vi "SWERVE_DRIVE_BEGIN.vi"(8 "error in (no error)":errorcluster) -> (0 "error out":errorcluster, 1 "Init Gyro Value":dbl, 2 "Swerve Module Pos":T1[](array[typedef]) {"Angle"."SIN" format="%13.4f"; "Angle"."COS" format="%13.4f"; "Angle"."VALUE" format="%13.4f"}, 3 "SWERVE_DRIVE_KINEMATICS":T3 {"SavedModuleStates"."Angle"."SIN" format="%13.4f"; "SavedModuleStates"."Angle"."COS" format="%13.4f"; "SavedModuleStates"."Angle"."VALUE" format="%13.4f"; "PrevCoR"."Y" format="%14.3f"; "PrevCoR"."X" format="%14.3f"; "Modules"."Y" format="%14.3f"; "Modules"."X" format="%14.3f"})   [LabVIEW 2019]
uses:
  <vilib>/Rock Robotics/WPI/ThirdParty/JAS_Junk/TrajLib/TypeDef/SWERVE_DRIVE_KINEMATICS.ctl
  <vilib>/Analysis/Matrix/Datatypes/RealMatrix.ctl
  <vilib>/Rock Robotics/WPI/ThirdParty/JAS_Junk/TrajLib/TypeDef/TRANSLATION2D.ctl
  <vilib>/Rock Robotics/WPI/ThirdParty/JAS_Junk/TrajLib/TypeDef/SWERVE_DRIVE_MODULE_STATE.ctl
  <vilib>/Rock Robotics/WPI/ThirdParty/JAS_Junk/TrajLib/TypeDef/ROTATION2D.ctl
  <vilib>/Rock Robotics/SystemInterfaces/AI/FPGA_AIGyroChannel.ctl
  <vilib>/Rock Robotics/SystemInterfaces/DIO/FPGA_DIOPWMChannel.ctl
  <vilib>/Rock Robotics/SystemInterfaces/DIO/FPGA_DIOChannel.ctl
  <vilib>/Rock Robotics/WPI/Gyro/WPI_GyroAnalogOpen.vi
  <vilib>/Rock Robotics/WPI/ThirdParty/JAS_Junk/TrajLib/Trajectory_Library.lvlib
  <vilib>/Analysis/Matrix/NI_Matrix.lvlib
  <vilib>/Rock Robotics/WPI/ThirdParty/JAS_Junk/TrajLib/TypeDef/SWERVE_DRIVE_MODULE_POSITION.ctl
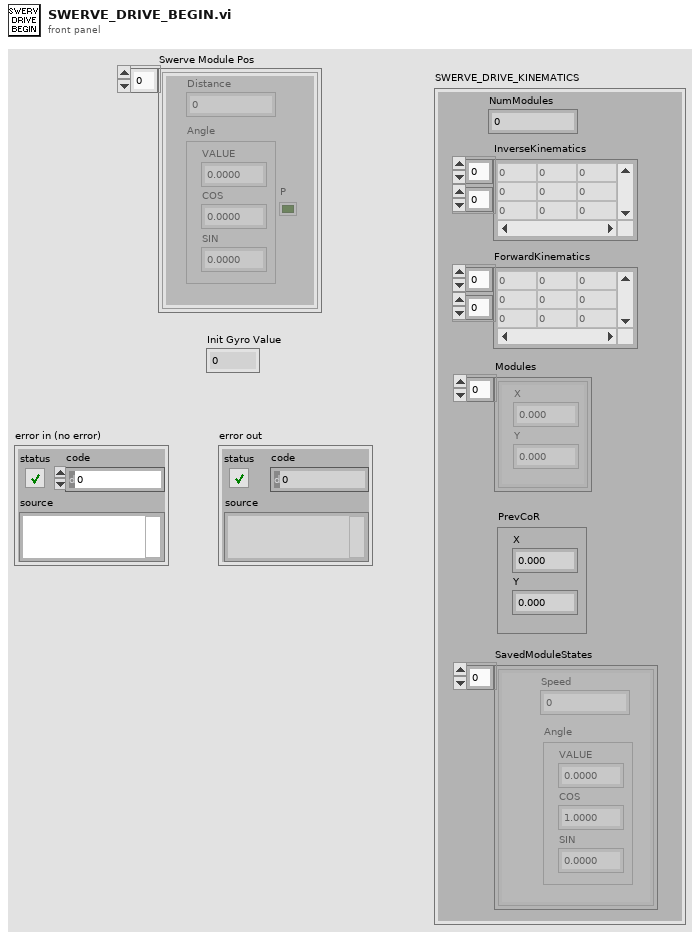
[diagram p1: front panel]
types:
  T1 = typedef "Trajectory_Library.lvlib/SWERVE_DRIVE_MODULE_POSITION.ctl" = cluster{"Distance":dbl, "Angle":T2, "P":bool}
  T2 = typedef "Trajectory_Library.lvlib/ROTATION2D.ctl" = cluster{"VALUE":dbl, "COS":dbl, "SIN":dbl}
  T3 = typedef "Trajectory_Library.lvlib/SWERVE_DRIVE_KINEMATICS.ctl" = cluster{"NumModules":i32, "InverseKinematics":T4, "ForwardKinematics":T4, "Modules":T5[], "PrevCoR":T5, "SavedModuleStates":T6[]}
  T4 = typedef "NI_Matrix.lvlib/RealMatrix.ctl" = dbl[][]
  T5 = typedef "Trajectory_Library.lvlib/TRANSLATION2D.ctl" = cluster{"X":dbl, "Y":dbl}
  T6 = typedef "Trajectory_Library.lvlib/SWERVE_DRIVE_MODULE_STATE.ctl" = cluster{"Speed":dbl, "Angle":T2}
  T7 = typedef "FPGA_DIOChannel.ctl" = enum8{"DIO 0", "DIO 1", "DIO 2", "DIO 3", "DIO 4", "DIO 5", "DIO 6", "DIO 7", "DIO 8", "DIO 9", "DIO MXP 0", "DIO MXP 1", "DIO MXP 2", "DIO MXP 3", "DIO MXP 4", "DIO MXP 5", "DIO MXP 6", "DIO MXP 7", "DIO MXP 8", "DIO MXP 9", "DIO MXP 10", "DIO MXP 11", "DIO MXP 12", "DIO MXP 13", "DIO MXP 14", "DIO MXP 15", "SPI Port CS1", "SPI Port CS2", "SPI Port CS3", "SPI Port MISO", "SPI Port MOSI", "Invalid"}
  T8 = typedef "FPGA_DIOPWMChannel.ctl" = enum8{"PWM 0", "PWM 1", "PWM 2", "PWM 3", "PWM 4", "PWM 5", "PWM 6", "PWM 7", "PWM 8", "PWM 9", "PWM MXP 0", "PWM MXP 1", "PWM MXP 2", "PWM MXP 3", "PWM MXP 4", "PWM MXP 5", "PWM MXP 6", "PWM MXP 7", "PWM MXP 8", "PWM MXP 9", "Invalid"}
  T9 = typedef "FPGA_AIGyroChannel.ctl" = enum8{"AI 0", "AI 1", "Invalid"}
  T10 = typedef "WPI_GyroDevRef.ctl" = cluster{"DevStatus":errorcluster, "Analog Channel":T11, "Gain (VoltsPerDegree/Second)":dbl, "Gyro Type":enum16{"Analog", "XRS450"}, "Handle":i32, "SPI Bus":T12, "Device Found":bool, "Sample Rate":dbl, "Calibrate On Open":bool, "Offset":dbl}
  T11 = typedef "FPGA_AIChannel.ctl" = enum8{"AI 0", "AI 1", "AI 2", "AI 3", "AI MXP 0", "AI MXP 1", "AI MXP 2", "AI MXP 3", "Invalid"}
  T12 = typedef "spi_bus.ctl" = enum16{"SPI On-Board, CS0", "SPI On-Board, CS1", "SPI On-Board, CS2", "SPI On-Board, CS3", "SPI MXP", "Invalid"}
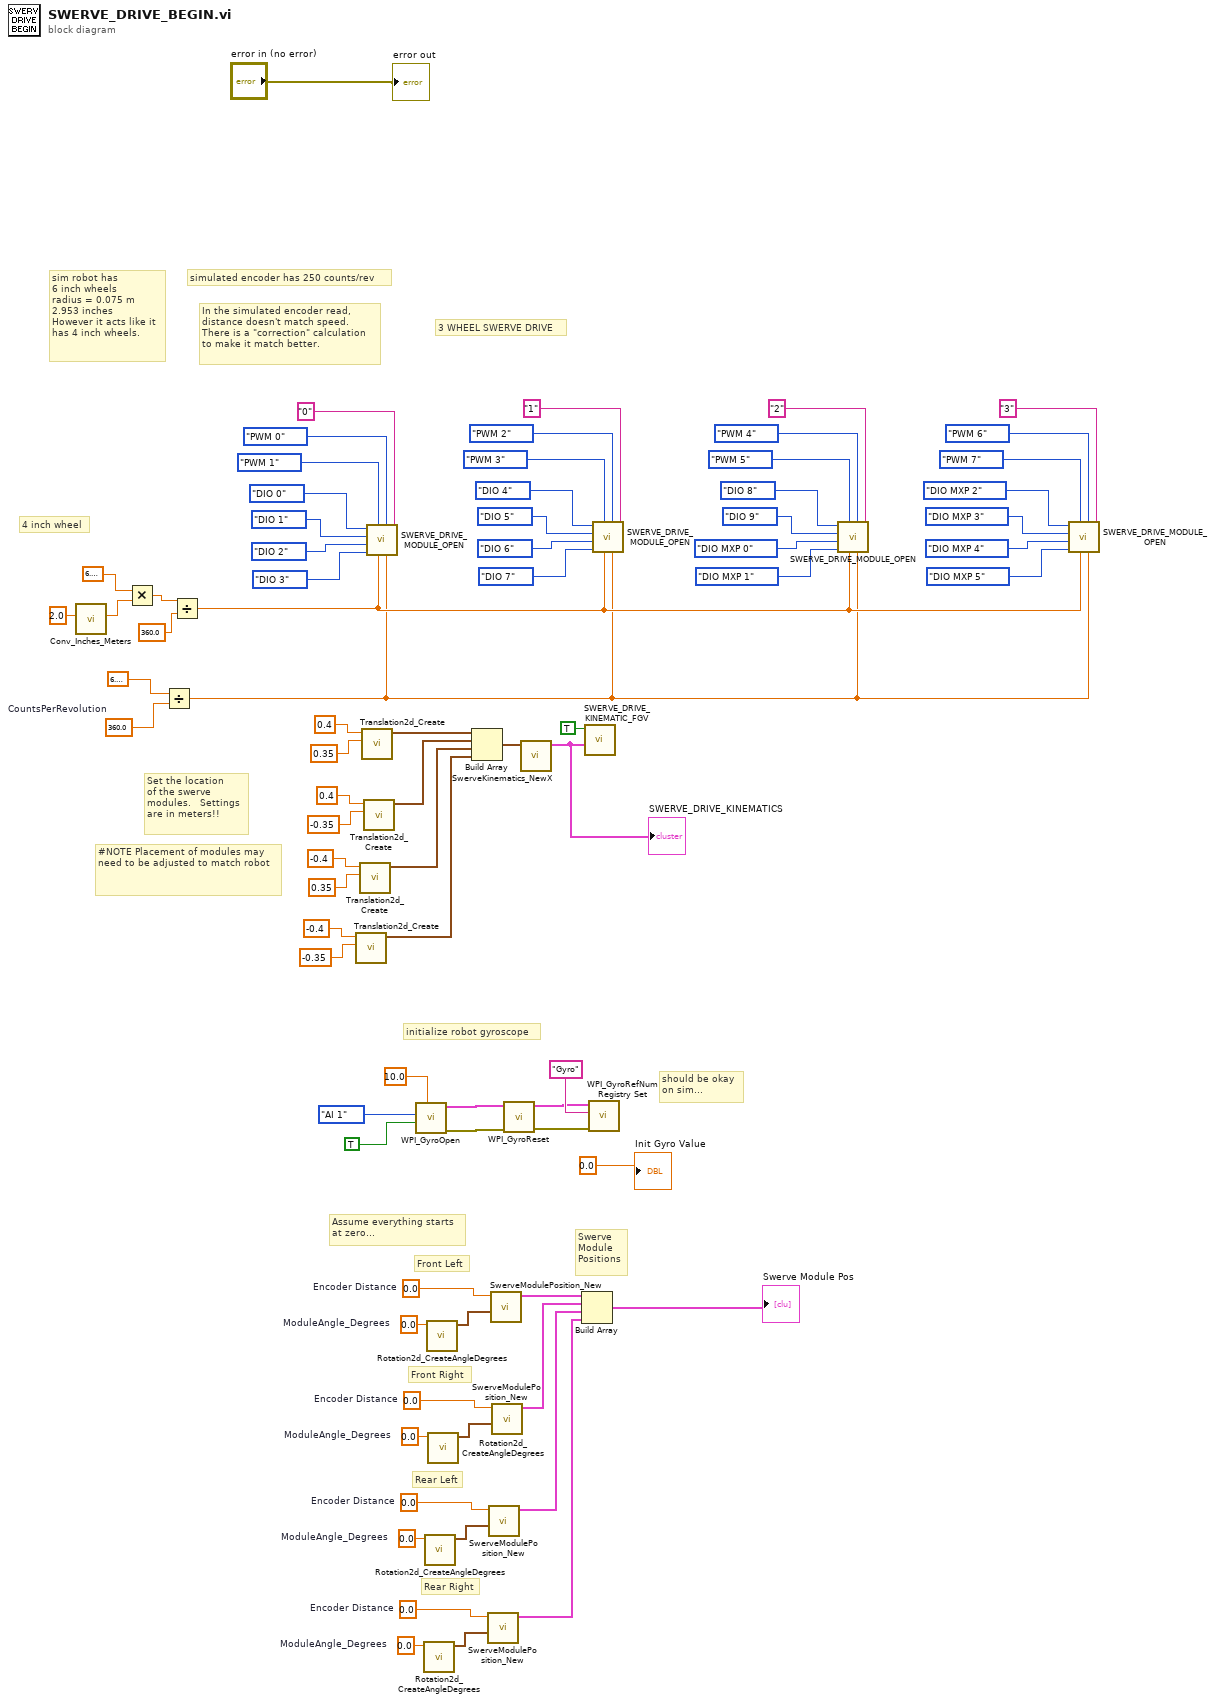
[diagram p0: block diagram]
diagram:
  w19 = 0.0  # ModuleAngle_Degrees
  w17 = 0.0  # Encoder Distance
  w16 = 0.0  # ModuleAngle_Degrees
  w14 = 0.0  # Encoder Distance
  w13 = 0.0  # ModuleAngle_Degrees
  w11 = 0.0  # Encoder Distance
  w9 = 0.0  # ModuleAngle_Degrees
  w7 = 0.0  # Encoder Distance
  w39 = 360.0  # CountsPerRevolution
  # "Assume everything starts\nat zero..."
  # "Front Left"
  # "Swerve\nModule\nPositions"
  # "Rear Right"
  # "Rear Left"
  # "Front Right"
  # "#NOTE Placement of modules may need to be adjusted to match robot"
  # "should be okay\non sim..."
  # "Set the location\nof the swerve \nmodules.   Settings\nare in meters!!"
  # "4 inch wheel"
  # "3 WHEEL SWERVE DRIVE"
  # "initialize robot gyroscope"
  # "In the simulated encoder read,\ndistance doesn't match speed.\nThere is a \"correction\" calculation\nto make it match better."
  # "simulated encoder has 250 counts/rev"
  # "sim robot has\n6 inch wheels\nradius = 0.075 m\n2.953 inches\nHowever it acts like it\nhas 4 inch wheels."
  n1 = call <vilib>:"Conv_Inches_Meters.vi"("INCH"=2.0) -> ("Meters"=w66:dbl)  [unwired: 10 in]
  n2 = Multiply(x=6.283185307179586, y=w66) -> (x*y=w25:dbl)
  n3 = Divide(x=6.283185307179586, y=w39) -> (x/y=w75:dbl)
  n4 = Divide(x=w25, y=360.0) -> (x/y=w76:dbl)
  n5 = call <vilib>:"Translation2d_Create.vi"("Y"=-0.35, "X"=-0.4) -> ("TRANSLATION"=w79:T5)  [unwired: 9 in]
  n6 = call <vilib>:"Translation2d_Create.vi"("Y"=0.35, "X"=-0.4) -> ("TRANSLATION"=w62:T5)  [unwired: 9 in]
  n7 = call <vilib>:"Translation2d_Create.vi"("Y"=0.35, "X"=0.4) -> ("TRANSLATION"=w60:T5)  [unwired: 9 in]
  n8 = call <vilib>:"Translation2d_Create.vi"("Y"=-0.35, "X"=0.4) -> ("TRANSLATION"=w61:T5)  [unwired: 9 in]
  n9 = call "SWERVE_DRIVE_MODULE_OPEN.vi"("NameSuffix"="0", "RadiansPerCount"=w75, "Drive PWM Channel"=FPGA_DIOPWMChannel."PWM 0", "DistancePerCount"=w76, "Swerve PWM Channel"=FPGA_DIOPWMChannel."PWM 1", "Swerve B Channel"=FPGA_DIOChannel."DIO 3", "Swerver A Channel"=FPGA_DIOChannel."DIO 2", "Drive B Channel"=FPGA_DIOChannel."DIO 1", "Drive A channel"=FPGA_DIOChannel."DIO 0") -> ()  [unwired: 3 in]
  n10 = call-poly <vilib>:"WPI_GyroOpen.vi"("Calibration Time (s)"=10.0, "Calibrate On Open"=TRUE, "Analog Channel"=FPGA_AIGyroChannel."AI 1") -> ("error out"=w4:errorcluster, "GyroDevRef"=w5:T10)  [unwired: 6 in, 1 out]
  n11 = call <vilib>:"Rotation2d_CreateAngleDegrees.vi"("Angle_Degrees"=w19) -> ("ROTATION"=w18:T2)  [unwired: 10 in]
  n12 = call <vilib>:"Rotation2d_CreateAngleDegrees.vi"("Angle_Degrees"=w16) -> ("ROTATION"=w15:T2)  [unwired: 10 in]
  n13 = call <vilib>:"Rotation2d_CreateAngleDegrees.vi"("Angle_Degrees"=w9) -> ("ROTATION"=w8:T2)  [unwired: 10 in]
  n14 = call <vilib>:"Rotation2d_CreateAngleDegrees.vi"("Angle_Degrees"=w13) -> ("ROTATION"=w12:T2)  [unwired: 10 in]
  n15 = Build Array(w60, w61, w62, w79) -> (w63:T5[])
  n16 = call <vilib>:"SwerveModulePosition_New.vi"("ROTATION"=w18, "Distance"=w17) -> ("SWERVE_DRIVE_MODULE_POSITION"=w22:T1)  [unwired: 9 in]
  n17 = call <vilib>:"SwerveModulePosition_New.vi"("ROTATION"=w15, "Distance"=w14) -> ("SWERVE_DRIVE_MODULE_POSITION"=w21:T1)  [unwired: 9 in]
  n18 = call <vilib>:"SwerveModulePosition_New.vi"("ROTATION"=w8, "Distance"=w7) -> ("SWERVE_DRIVE_MODULE_POSITION"=w10:T1)  [unwired: 9 in]
  n19 = call <vilib>:"SwerveModulePosition_New.vi"("ROTATION"=w12, "Distance"=w11) -> ("SWERVE_DRIVE_MODULE_POSITION"=w20:T1)  [unwired: 9 in]
  n20 = call <vilib>:"WPI_GyroReset.vi"("error in (no error)"=w4, "GyroDevRef"=w5) -> ("error out"=w2:errorcluster, "GyroDevRef"=w3:T10)  [unwired: 8 in]
  n21 = call <vilib>:"SwerveKinematics_NewX.vi"("Wheels"=w63) -> ("SWERVE_DRIVE_KINEMATICS"=w65:T3)  [unwired: 10 in]
  "SWERVE_DRIVE_KINEMATICS" <- w65
  n22 = Build Array(w10, w20, w21, w22) -> (→"Swerve Module Pos":T1[])
  n23 = call "SWERVE_DRIVE_KINEMATIC_FGV.vi"("in SWERVE_DRIVE_KINEMATICS"=w65, "WRITE"=TRUE) -> ()  [unwired: 9 in, 1 out]
  n24 = call <vilib>:"WPI_GyroRefNum Registry Set.vi"("error in (no error)"=w2, "refnum name"="Gyro", "GyroDevRef"=w3) -> ()  [unwired: 7 in, 2 out]
  n25 = call "SWERVE_DRIVE_MODULE_OPEN.vi"("NameSuffix"="1", "RadiansPerCount"=w75, "Drive PWM Channel"=FPGA_DIOPWMChannel."PWM 2", "DistancePerCount"=w76, "Swerve PWM Channel"=FPGA_DIOPWMChannel."PWM 3", "Swerve B Channel"=FPGA_DIOChannel."DIO 7", "Swerver A Channel"=FPGA_DIOChannel."DIO 6", "Drive B Channel"=FPGA_DIOChannel."DIO 5", "Drive A channel"=FPGA_DIOChannel."DIO 4") -> ()  [unwired: 3 in]
  n26 = call "SWERVE_DRIVE_MODULE_OPEN.vi"("NameSuffix"="2", "RadiansPerCount"=w75, "Drive PWM Channel"=FPGA_DIOPWMChannel."PWM 4", "DistancePerCount"=w76, "Swerve PWM Channel"=FPGA_DIOPWMChannel."PWM 5", "Swerve B Channel"=FPGA_DIOChannel."DIO MXP 1", "Swerver A Channel"=FPGA_DIOChannel."DIO MXP 0", "Drive B Channel"=FPGA_DIOChannel."DIO 9", "Drive A channel"=FPGA_DIOChannel."DIO 8") -> ()  [unwired: 3 in]
  n27 = call "SWERVE_DRIVE_MODULE_OPEN.vi"("NameSuffix"="3", "RadiansPerCount"=w75, "Drive PWM Channel"=FPGA_DIOPWMChannel."PWM 6", "DistancePerCount"=w76, "Swerve PWM Channel"=FPGA_DIOPWMChannel."PWM 7", "Swerve B Channel"=FPGA_DIOChannel."DIO MXP 5", "Swerver A Channel"=FPGA_DIOChannel."DIO MXP 4", "Drive B Channel"=FPGA_DIOChannel."DIO MXP 3", "Drive A channel"=FPGA_DIOChannel."DIO MXP 2") -> ()  [unwired: 3 in]
  "error out" <- "error in (no error)"
  "Init Gyro Value" <- 0.0
